vi "Build Bar Plot.vi"(0 "XYGraph in":refnum<vi>, 5 "Picture Ref":refnum<vi>, 7 "Y Scale Label":string, 9 "Labels":string[](array[string]), 11 "Error In":errorcluster) -> (4 "Picture":picture, 15 "Error Out":errorcluster)   [LabVIEW 2020]
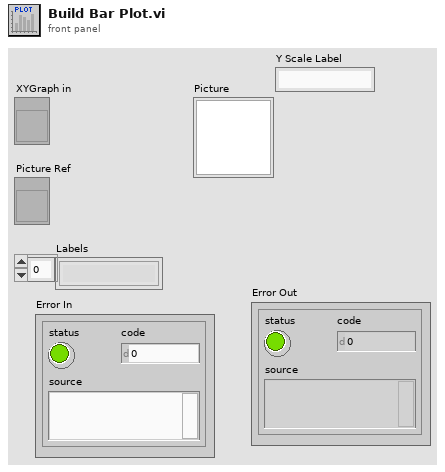
[diagram p1: front panel]
types:
  T1 = enum16{"None", "Stacked", "Clockwise", "Counterclockwise"}
  T2 = cluster{"horizontal":enum16{"left", "center", "right"}, "vertical":enum16{"top", "center", "bottom"}}
  T3 = enum16{"User-specified Font", "Application Font", "System Font", "Dialog Font"}
  T4 = typedef "LVBoundsTypeDef.ctl" = cluster{"Width":u32, "Height":u32}
  T5 = cluster{"Font Name:":string, "Size":i16, "Strikeout?":bool, "Italic?":bool, "Underline?":bool, "Outline?":bool, "Shadow?":bool, "Bold?":bool}
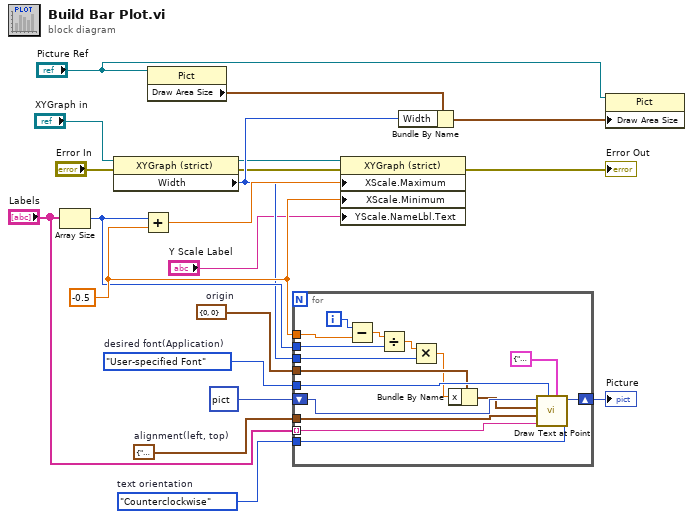
[diagram p0: block diagram]
diagram:
  w19 = T1."Counterclockwise"  # text orientation
  w17 = T2 {"horizontal"=enum."center", "vertical"=enum."top"}  # alignment(left, top)
  w14 = -0.5 ("X Scale.Range:Minimum")
  w16 = T3."User-specified Font"  # desired font(Application)
  w18 = cluster{"x":i16, "y":i16} {"x"=0, "y"=0}  # origin
  n1 = Array Size(array="Labels") -> (size(s)=w9:i32)
  n2 = property on="Property Node" class="XYGraph (strict)"(reference="XYGraph in", error in="Error In") -> (reference out=w4:refnum<vi>, error out=w3:errorcluster, "Width"=w8:u32)
  n3 = Add(x=w9, y=w14) -> (x+y=w10:dbl)
  n4 = property on="Property Node" class="Pict"(reference="Picture Ref") -> ("Draw Area Size"=w11:T4)  [unwired: 1 in, 2 out]
  n5 = for {
    tunnel: "Labels" -> [w34] mode=indexing
    shift-right: [w35] -> w13
    shift-left: picture data[5B] ("Picture") -> [w36]
    tunnel: w16 -> [w33]
    tunnel: w17 -> [w32]
    tunnel: w18 -> [w31]
    tunnel: w14 -> [w27]
    tunnel: w9 -> [w29]
    tunnel: w8 -> [w24]
    tunnel: w19 -> [w22]
    i -> [w28]
    n6 = Subtract(x=w28, y=w27) -> (x-y=w26:dbl)
    n7 = Divide(x=w26, y=w29) -> (x/y=w25:dbl)
    n8 = Multiply(x=w25, y=w24) -> (x*y=w23:dbl)
    n9 = Bundle By Name(cluster=w31, "x"=w23) -> (w30:cluster{"x":i16, "y":i16})
    n10 = call <vilib>:"Draw Text at Point.vi"("text orientation"=w22, "[user-specified font]"=T5 {"Font Name:"="Application Font", "Size"=15, "Strikeout?"=FALSE, "Italic?"=FALSE, "Underline?"=FALSE, "Outline?"=FALSE, "Shadow?"=FALSE, "Bold?"=TRUE}, "desired font(Application)"=w33, "text"=w34, "alignment(left, top)"=w32, "origin"=w30, "picture"=w36) -> ("new picture"=w35:picture)  [unwired: 3 in, 1 out]
  }
  "Picture" <- w13
  n11 = property on="Property Node" class="XYGraph (strict)"(reference=w4, error in=w3, "XScale.Maximum"=w10, "XScale.Minimum"=w14, "YScale.NameLbl.Text"="Y Scale Label") -> (error out=→"Error Out":errorcluster)  [unwired: 1 out]
  n12 = Bundle By Name(cluster=w11, "Width"=w8) -> (w12:T4)
  n13 = property on="Property Node" class="Pict"(reference="Picture Ref", "Draw Area Size"=w12) -> ()  [unwired: 1 in, 2 out]
